vi "(Depricated) Launch Interlock.vi"(8 "error in (no error)":errorcluster, 10 "Interlocks.lvlib:Interlock.lvclass":refnum<class "Interlock.lvclass">, 11 "Interlock Chain in":refnum<class "Interlock Chain.lvclass">) -> (0 "error out":errorcluster, 3 "Interlock Chain out":refnum<class "Interlock Chain.lvclass">)   [LabVIEW 2015, in "Interlocks.lvlib" / "Interlock Chain.lvclass"]
uses:
  Interlock Chain.lvclass
  Interlock/Interlock.lvclass
  <vilib>/ActorFramework/Actor/Actor.lvclass
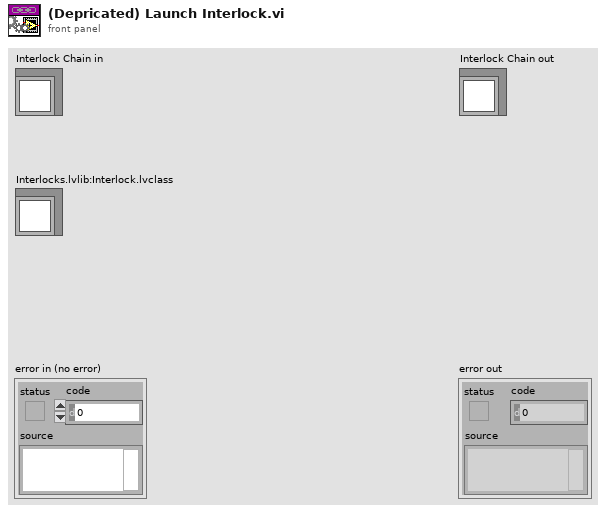
[diagram p1: front panel]
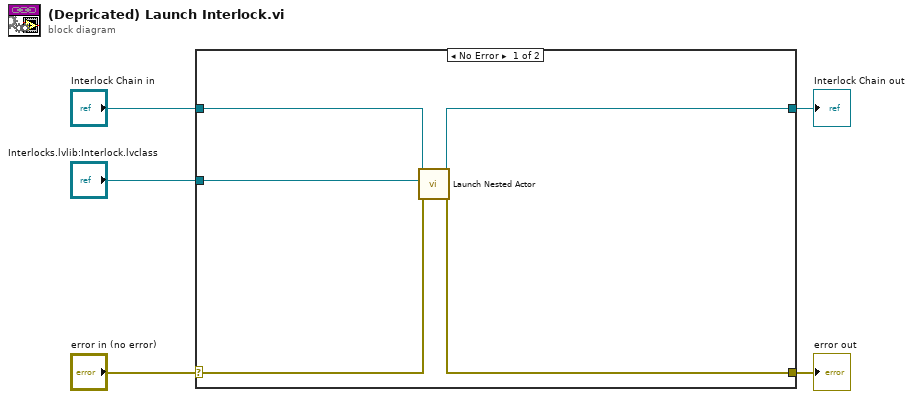
[diagram p0: block diagram]
diagram:
  n1 = case shown="No Error" "error in (no error)" {
    selector: "error in (no error)" -> [w7 w12]
    tunnel: [w6 w12] -> w4
    tunnel: [w8 w11] -> w2
    tunnel: "Interlock Chain in" -> [w9 w11]
    tunnel: "Interlocks.lvlib:Interlock.lvclass" -> [w10 _]
    frame No Error {
      n2 = call <vilib>:"Launch Nested Actor.vi"("error in (no error)"=w7, "Nested Actor"=w10, "Caller Actor in"=w9) -> ("error out"=w6:errorcluster, "Caller Actor out"=w8:refnum<class "Interlock Chain.lvclass">)  [unwired: 6 in, 1 out]
    }
    frame Error {
    }
  }
  "error out" <- w4
  "Interlock Chain out" <- w2
